vi "Project.vi"() -> ()   [LabVIEW 2020]
uses:
  <userlib>/_OpenG.lib/comparison/comparison.llb/DBL Changed__ogtk.vi
  <vilib>/Simulation/Implementation/XNodeFramework/SimXNode/SimX.xnode
  <vilib>/Simulation/Model Libraries/PID/SIM PID.vi
  <vilib>/Simulation/Model Libraries/PID/SIM PID (Academic).vi
  <vilib>/Simulation/Implementation/Shared/SIMSCR Execution Mode.ctl
  <vilib>/Simulation/Scripting/Companion Diagram/SimConfigNode/_simSolvers.ctl
  <vilib>/Simulation/Scripting/Companion Diagram/SimConfigNode/SimParams.ctl
  <vilib>/Simulation/Scripting/Companion Diagram/SimConfigNode/SimDog.xnode
panel:
  in  "stop":bool
  in  "Max Temperature (F)":dbl=40.0
  out "System Humidity":dbl[](graph)
  out "System Temperature":dbl[](graph)
  out "Light Status":bool
  in  "Light End":timestamp=timestamp(7200 s since 1904-01-01) format="%<%I:%M %p>T"
  in  "Light Start Stamp":timestamp=timestamp(-43200 s since 1904-01-01) format="%<%I:%M %p>T"
  in  "Desired Water Level":dbl(slide)=8.061224489795919 scale=0.0..10.0
  in  "Max Humidity (%)":dbl=40.0
  out "Environment Temperature (F)":dbl=68.0
  out "Environment Humidity (%)":dbl=35.0
  out "System Humidity (%)":dbl
  out "System Temperature (F)":dbl
  out "Water Level":dbl(slide) scale=0.0..10.0
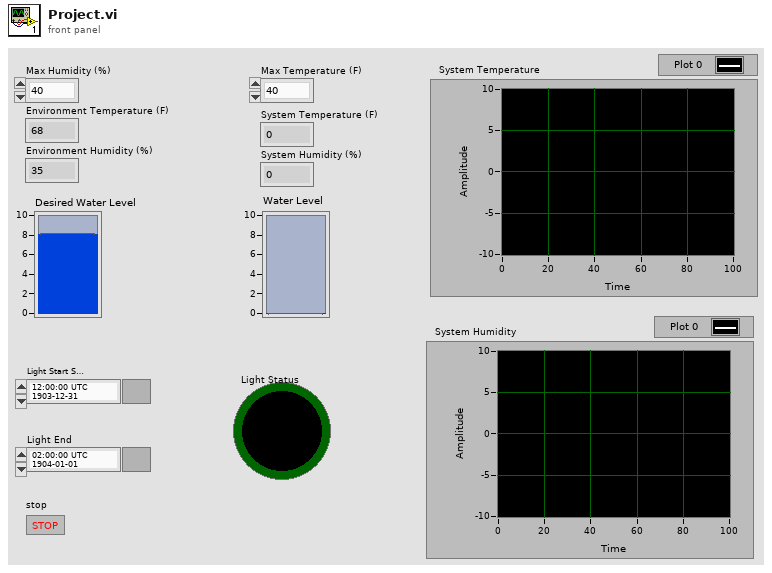
[diagram p1: front panel]
types:
  T1 = enum16{"Simulate to Completion", "Single Time-Step Simulation (Fixed Step Only)"}
  T2 = typedef "SimParams.ctl" = cluster{"Initial Time (s)":dbl, "Final Time (s)":dbl, "Step Size (s)":dbl, "ODE Solver":T3, "Minimum Step Size (s)":dbl, "Maximum Step Size (s)":dbl, "Relative Tolerance":dbl, "Absolute Tolerance":dbl, "Software Timing":bool, "Initial Step Size (s)":dbl, "Automatic Fixed Step Size?":bool, "Automatic Discrete Step Size?":bool, "Discrete Step Size (s)":dbl, "Calculate using Time Step":bool, "Solver Wired?":bool, "Prev.Frm.Expected End":u64, "Prev.Frm.Actual End":u64, "Prev.Frm.Finished Late?":bool, "Prev.Iter.Expected End":u64, "Prev.Iter.Actual End":u64, "Prev.Iter.Finished Late?":bool, "Expected Iteration Start":u64, "Actual Iteration Start":u64, "Expected Frame Start":u64, "Actual Frame Start":u64, "Source Name":string, "Name":string, "Period":i64, "Deadline":i64, "Offset":i64, "Start":i64, "Priority":i32, "Timeout":i32, "Processor":i32, "Mode":enum32{"No Change", "Process missed periods, maintain original phase", "Discard missed periods, maintain original phase", "Process missed periods, ignore original phase", "Discard missed periods, ignore original phase"}, "Wakeup reason":enum32{"Normal", "Aborted", "Asynchronous wakeup", "Timing source error", "Timed loop error", "Timeout"}, "Error":errorcluster, "Source Type":string, "Secondary Source Type":string, "Global End Time":u64, "Global Start Time":u64, "Full Solver Reset":bool, "Execution Mode":T4, "Nan/Inf Check":bool, "Custom Solver Library":string, "Solver Is Variable":bool, "custom solver name":string, "Signal Collection Decimation":u32}
  T3 = typedef "_simSolvers.ctl" = enum16{"Runge-Kutta 1 (Euler)", "Runge-Kutta 2", "Runge-Kutta 3", "Runge-Kutta 4", "Runge-Kutta 23 (variable)", "Runge-Kutta 45 (variable)", "BDF (variable)", "Adams-Moulton (variable)", "Rosenbrock (variable)", "Discrete States Only", "SDIRK 4 (variable)", "Radau 5 (variable)", "Radau 9 (variable)", "Radau 13 (variable)", "Radau [Variable Order] (variable)", "Gear's Method (variable)", "Linearizer", "State Query", "Trim Eval", "Custom Solver"}
  T4 = typedef "SIMSCR Execution Mode.ctl" = enum16{"Simulate to Completion", "Single Time-Step Simulation (Fixed Step Only)"}
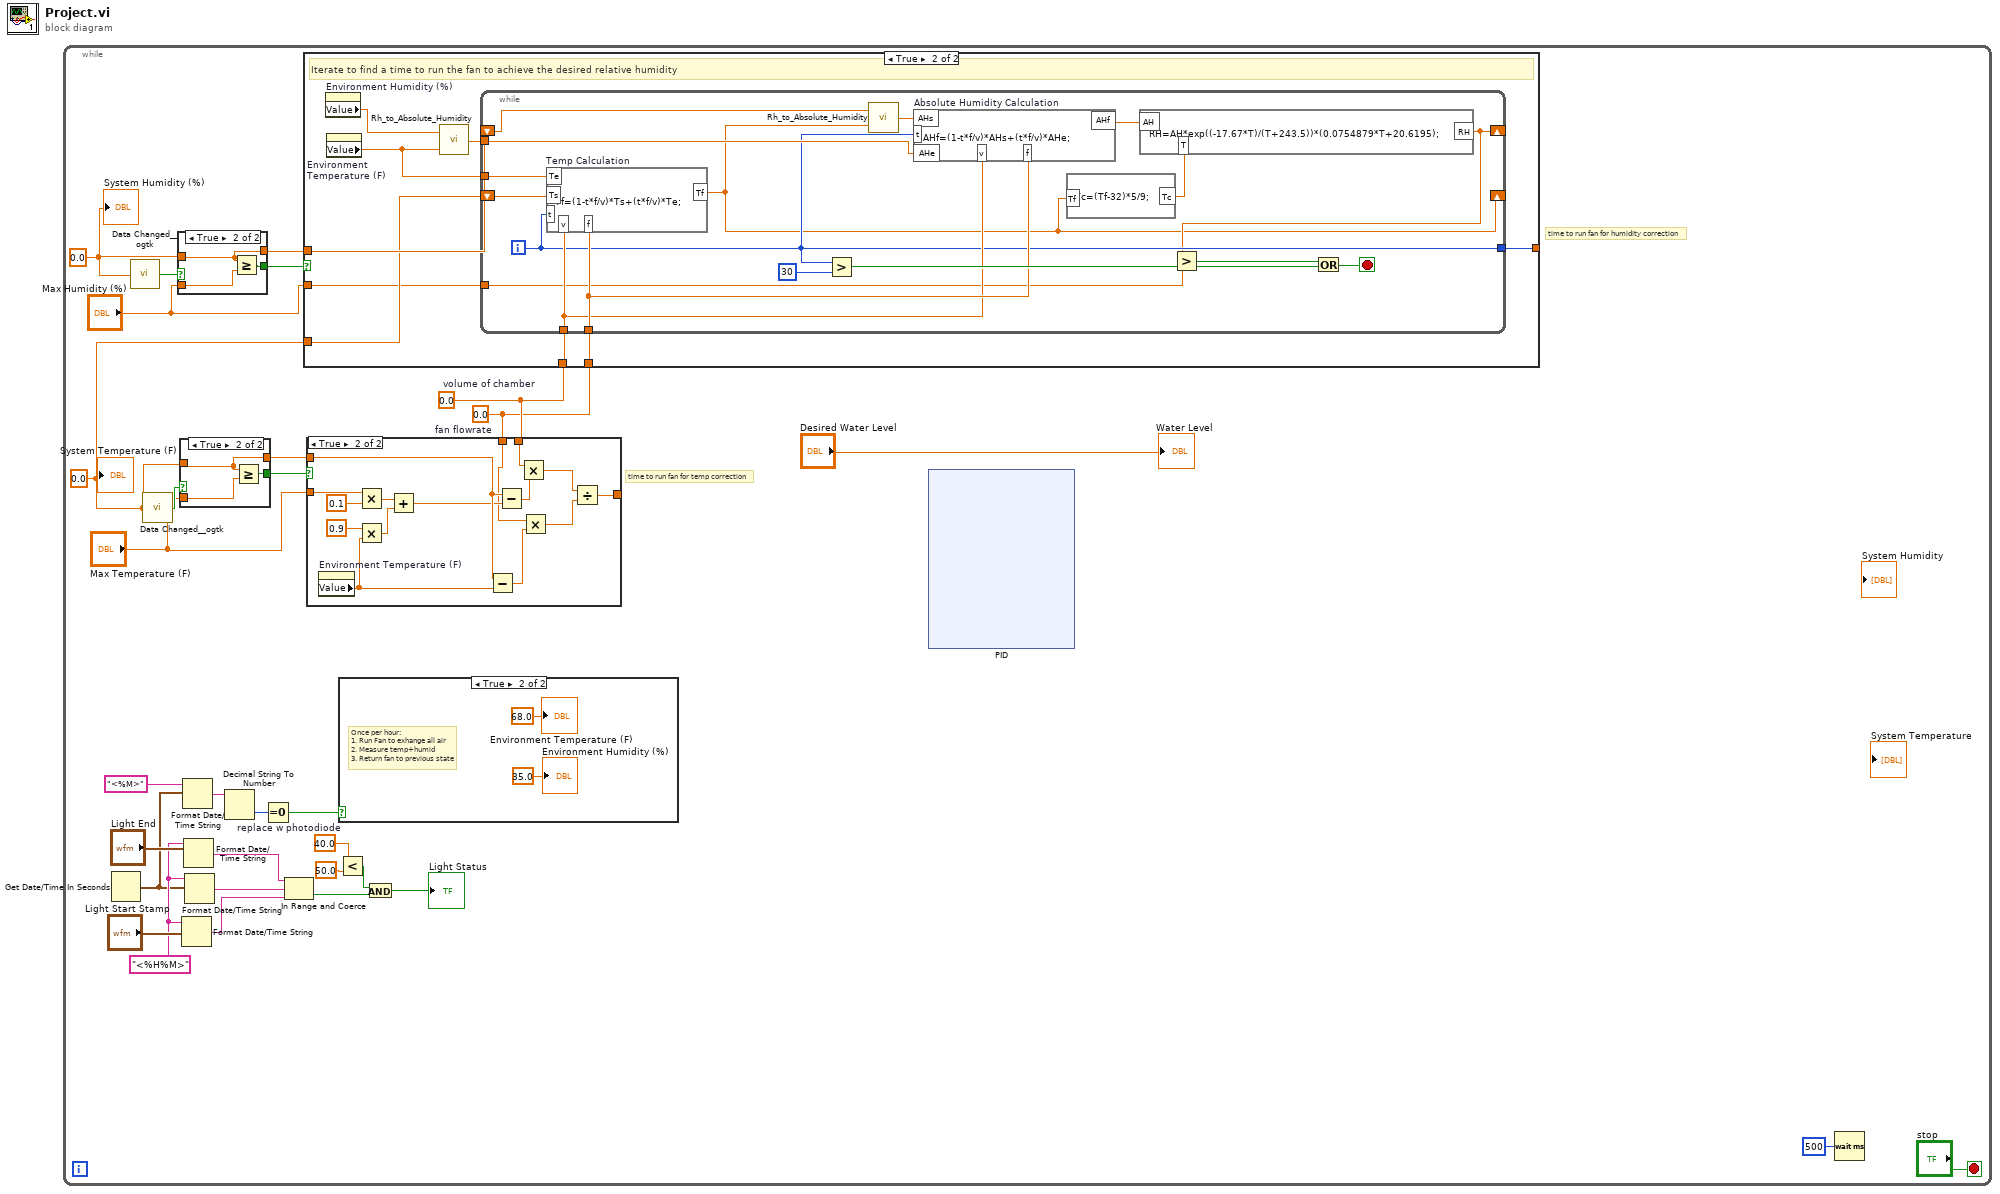
[diagram p0: block diagram]
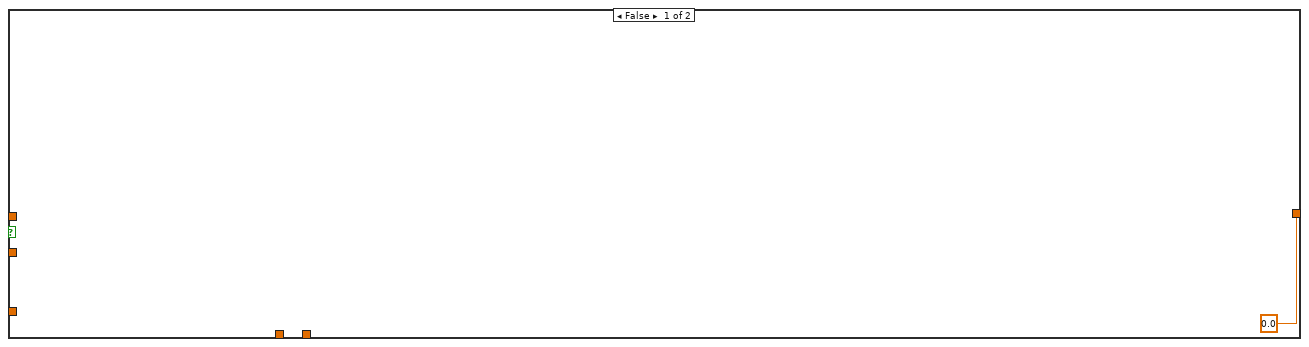
[diagram p2: hidden frame]
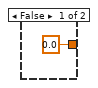
[diagram p3: hidden frame]
diagram:
  n1 = while {
    stop <- "stop" stop-if-true
    w2 = 0.0  # volume of chamber
    w1 = 0.0  # fan flowrate
    w3 = 0.0 ("System Humidity (%)")
    w12 = 0.0 ("System Humidity (%)")
    w19 = 40.0  # replace w photodiode
    w24 = "<%H%M>"
    # "time to run fan for humidity correction"
    # "time to run fan for temp correction"
    n2 = Get Date/Time In Seconds() -> (seconds since 1Jan1904=w18:timestamp)
    n3 = call-poly <userlib>:"Data Changed__ogtk.vi"("DBL"=w12) -> ("Changed"=w13:bool)
    n4 = call-poly <userlib>:"Data Changed__ogtk.vi"("DBL"=w3) -> ("Changed"=w11:bool)
    n5 = case shown="True" w13 {
      selector: w13 -> [w107 _]
      tunnel: w12 -> [w106 w109]
      tunnel: [w107 w110] -> w6
      tunnel: [w106 w109] -> w4
      tunnel: "Max Humidity (%)" -> [_ w108]
      frame False {
      }
      frame True {
        n6 = Greater Or Equal?(x=w109, y=w108) -> (x >= y?=w110:bool)
      }
    }
    n7 = case shown="True" w11 {
      selector: w11 -> [w102 _]
      tunnel: w3 -> [w101 w104]
      tunnel: [w102 w105] -> w10
      tunnel: [w101 w104] -> w9
      tunnel: "Max Temperature (F)" -> [_ w103]
      frame False {
      }
      frame True {
        n8 = Greater Or Equal?(x=w104, y=w103) -> (x >= y?=w105:bool)
      }
    }
    n9 = Format Date/Time String(time format string (%c)=w24, seconds (now)="Light Start Stamp") -> (date/time string=w27:string)  [unwired: 1 in]
    n10 = Format Date/Time String(time format string (%c)="<%M>", seconds (now)=w18) -> (date/time string=w17:string)  [unwired: 1 in]
    n11 = Format Date/Time String(time format string (%c)=w24, seconds (now)="Light End") -> (date/time string=w28:string)  [unwired: 1 in]
    n12 = Format Date/Time String(time format string (%c)=w24, seconds (now)=w18) -> (date/time string=w26:string)  [unwired: 1 in]
    n13 = Decimal String To Number(string=w17) -> (number=w16:i32)  [unwired: 2 in, 1 out]
    n14 = Equal To 0?(x=w16) -> (x = 0?=w14:bool)
    n15 = In Range and Coerce(upper limit=w28, x=w26, lower limit=w27) -> (In Range?=w23:bool)  [unwired: 1 out]
    n16 = case shown="True" w6 {
      tunnel: w4 -> [_ w67]
      tunnel: [0.0 w60] -> _
      tunnel: "Max Humidity (%)" -> [_ w59]
      tunnel: w3 -> [_ w66]
      tunnel: w2 -> [_ w64]
      tunnel: w1 -> [_ w63]
      frame False {
      }
      frame True {
        # "Iterate to find a time to run the fan to achieve the desired relative humidity"
        n17 = property on="Environment Humidity (%)" class="DigNum (strict)"() -> ("Value"=w62:dbl)  [unwired: 2 in, 2 out]
        n18 = property on="Environment Temperature (F)" class="DigNum (strict)"() -> ("Value"=w65:dbl)  [unwired: 2 in, 2 out]
        n19 = call "Rh_to_Absolute_Humidity.vi"("Temperature (F)"=w65, "Relative Humidity"=w62) -> ("Absolute Humidity"=w61:dbl)
        n20 = while {
          tunnel: w65 -> [w79]
          tunnel: w64 -> [w76]
          tunnel: w63 -> [w77]
          shift-right: [w69] -> _
          shift-left: w66 -> [w84]
          tunnel: w61 -> [w75]
          shift-right: [w72] -> _
          shift-left: w67 -> [w80]
          tunnel: [w74] -> w60
          tunnel: w59 -> [w71]
          i -> [w74]
          stop <- w83 stop-if-true
          n21 = formula code="Tf=(1-t*f/v)*Ts+(t*f/v)*Te;" "Temp Calculation"("Te"=w79, "Ts"=w84, "t"=w74, "v"=w76, "f"=w77) -> ("Tf"=w69:dbl)
          n22 = Greater?(x=w74, y=30) -> (0:w82:bool)
          n23 = call "Rh_to_Absolute_Humidity.vi"("Temperature (F)"=w69, "Relative Humidity"=w80) -> ("Absolute Humidity"=w78:dbl)
          n24 = formula code="AHf=(1-t*f/v)*AHs+(t*f/v)*AHe;" "Absolute Humidity Calculation"("AHs"=w78, "AHe"=w75, "v"=w76, "f"=w77, "t"=w74) -> ("AHf"=w73:dbl)
          n25 = formula code="Tc=(Tf-32)*5/9;"("Tf"=w69) -> ("Tc"=w68:dbl)
          n26 = formula code="RH=AH*exp((-17.67*T)/(T+243.5))*(0.0754879*T+20.6195);"("AH"=w73, "T"=w68) -> ("RH"=w72:dbl)
          n27 = Greater?(x=w72, y=w71) -> (0:w70:bool)
          n28 = Or(x=w70, y=w82) -> (x .or. y?=w83:bool)
        }
      }
    }
    n29 = case shown="True" w10 {
      tunnel: w9 -> [_ w95]
      tunnel: [0.0 w100] -> _
      tunnel: "Max Temperature (F)" -> [_ w94]
      tunnel: w1 -> [_ w87]
      tunnel: w2 -> [_ w86]
      frame False {
      }
      frame True {
        n30 = property on="Environment Temperature (F)" class="DigNum (strict)"() -> ("Value"=w93:dbl)  [unwired: 2 in, 2 out]
        n31 = Multiply(x=w94, y=0.1) -> (x*y=w90:dbl)
        n32 = Multiply(x=0.9, y=w93) -> (x*y=w89:dbl)
        n33 = Add(x=w90, y=w89) -> (x+y=w88:dbl)
        n34 = Subtract(x=w95, y=w93) -> (x-y=w97:dbl)
        n35 = Subtract(x=w95, y=w88) -> (x-y=w96:dbl)
        n36 = Multiply(x=w86, y=w96) -> (x*y=w98:dbl)
        n37 = Multiply(x=w87, y=w97) -> (x*y=w99:dbl)
        n38 = Divide(x=w98, y=w99) -> (x/y=w100:dbl)
      }
    }
    n39 = Less?(x=w19, y=50.0) -> (x < y?=w22:bool)
    n40 = case shown="True" w14 {
      frame False {
      }
      frame True {
        # "Once per hour:\n1. Run Fan to exhange all air\n2. Measure temp+humid\n3. Return fan to previous state"
        "Environment Temperature (F)" <- 68.0 ("Environment Temperature (F)")
        "Environment Humidity (%)" <- 35.0 ("Environment Humidity (%)")
      }
    }
    n41 = And(x=w22, y=w23) -> (x .and. y?=→"Light Status":bool)
    n42 = xnode "PID"() -> ()  [unwired: 3 in, 12 out]
    n43 = Wait (ms)(milliseconds to wait=u32 500) -> ()  [unwired: 1 out]
    "Water Level" <- "Desired Water Level"
    "System Temperature (F)" <- w3
    "System Humidity (%)" <- w12
  }
